vi "[FPGA] eHS Main (9039).vi"() -> ()   [LabVIEW 2017]
uses:
  <vilib>/OPAL-RT/eHS Toolkit/eHS Common/Controls/eHSx64 Gen3 Configuration.ctl
  <vilib>/OPAL-RT/Utilities Toolkit/Mapping/Input Mapping/FPGA/Controls/Input Mapping Configuration FIFO.ctl
  <vilib>/OPAL-RT/Utilities Toolkit/Mapping/Switch Mapping/FPGA/Controls/Switch Mapping Configuration FIFO.ctl
  <vilib>/OPAL-RT/Analog I-O Mapping & Conditioning Toolkit/AOMC/FPGA/Public/Controls/AOMC Configuration FIFO.ctl
  <vilib>/Platform/TimedLoop/XDataNode/timing_clust.ctl
  <vilib>/Platform/TimedLoop/XDataNode/nitl_modes.ctl
  <vilib>/Platform/TimedLoop/XDataNode/wakeup.ctl
  <vilib>/OPAL-RT/Analog I-O Mapping & Conditioning Toolkit/AIC/FPGA/Public/Controls/AIC Configuration FIFO.ctl
  <vilib>/OPAL-RT/FPGA Signal Generation Toolkit/Sinewave Generation/FPGA/Public/Controls/Sinewave Configuration FIFO.ctl
  <vilib>/OPAL-RT/FPGA Signal Generation Toolkit/SPWM Generation/FPGA/Public/Controls/SPWM Configuration FIFO.ctl
  <vilib>/OPAL-RT/FPGA Signal Generation Toolkit/PWM Generation/FPGA/Public/Controls/PWM Configuration FIFO.ctl
  <vilib>/OPAL-RT/Analog I-O Mapping & Conditioning Toolkit/AOMC/FPGA/Public/Controls/Input Sources.ctl
  <vilib>/OPAL-RT/Utilities Toolkit/Mapping/Input Mapping/FPGA/Controls/Sources/Input Sources - Parallelx32.ctl
  <vilib>/OPAL-RT/Utilities Toolkit/Mapping/Switch Mapping/FPGA/Controls/Sources/Switch Sources - Parallelx72.ctl
  <vilib>/rvi/Emulation/niFpgaGetClockAttributes.vi
  <vilib>/rvi/Emulation/niFpgaSctlEmulationGetInTimedLoop.vi
  <vilib>/rvi/Emulation/niFpgaEmulationReportErrorSimple.vi
  <vilib>/OPAL-RT/Utilities Toolkit/Mapping/Input Mapping/FPGA/SubVIs/Initialize/Initialize Input Mapping - Parallelx32.vi
  <vilib>/OPAL-RT/Utilities Toolkit/Mapping/Switch Mapping/FPGA/SubVIs/Initailize/Initialize Switch Mapping - Parallelx72.vi
  <vilib>/rvi/DataTransferAndStorage/Container/Common/niFpgaContainerExecOnDevCompGetState.vi
  <vilib>/rvi/Emulation/niFpgaEmulationIsFPGAContextNoSignature.vi
  <vilib>/rvi/DataTransferAndStorage/Container/Common/niFpgaContainerGetUniqueNameForEmu.vi
  <vilib>/rvi/Memory/Memory_Emulation/niFpgaMemoryEmulationCacheClearOnFirstRun.vi
  <vilib>/rvi/Memory/Memory_Emulation/nirvimemoryEmulationManagerCache_MakeExclusive.vi
  <vilib>/rvi/Memory/Memory_Emulation/niFpgaMemoryEmulationValidateCache.vi
  <vilib>/rvi/Memory/Memory_Emulation/nirvimemoryEmulationManagerCache_InsertValue.vi
  <vilib>/Utility/error.llb/Clear Errors.vi
  <vilib>/rvi/Memory/Memory_Emulation/nirvimemoryEmulationManagerCache_ReleaseExclusive.vi
  <vilib>/rvi/Memory/Memory_Emulation/nirvimemoryEmulationManagerCache_GetValue.vi
  <vilib>/rvi/Memory/Memory_Emulation/nirvimemoryEmulationManagerCache_SetValue.vi
  <vilib>/rvi/Emulation/niFpgaProcessEmulError.vi
  <vilib>/rvi/eio/common/nirviEmuTemplateMethod_errors.vi
  <vilib>/rvi/Emulation/niFpgaCriticalErrorInLSC.vi
  <vilib>/OPAL-RT/FPGA Signal Generation Toolkit/Sinewave Generation/FPGA/Private/Generators/Sinewave Generators (32-CH Parallel).vi
  <vilib>/OPAL-RT/FPGA Signal Generation Toolkit/SPWM Generation/FPGA/Private/Generators/SPWM Generators (12-CH Parallel).vi
  <vilib>/OPAL-RT/FPGA Signal Generation Toolkit/PWM Generation/FPGA/Private/Generators/PWM Generators (16-CH Parallel).vi
  <vilib>/OPAL-RT/Analog I-O Mapping & Conditioning Toolkit/AOMC/FPGA/Private/AO Mapping & Conditioning (FXP(20,5)).vi
  <vilib>/OPAL-RT/Analog I-O Mapping & Conditioning Toolkit/AIC/FPGA/Private/AI Conditioning FXP(20,5).vi
  <vilib>/OPAL-RT/eHS Toolkit/eHS FPGA/SubVIs/eHSx64 Gen3 Solver Core.vi
  <vilib>/OPAL-RT/Utilities Toolkit/Mapping/Switch Mapping/FPGA/SubVIs/Configure/Get Switch Mapping Configuration from Host - Parallelx72.vi
  <vilib>/OPAL-RT/Utilities Toolkit/Mapping/Input Mapping/FPGA/SubVIs/Configure/Get Input Mapping Configuration from Host - Parallelx32.vi
  <vilib>/OPAL-RT/Utilities Toolkit/Mapping/Switch Mapping/FPGA/SubVIs/Map/Map Switches - Parallelx72.vi
  <vilib>/OPAL-RT/Utilities Toolkit/Mapping/Input Mapping/FPGA/SubVIs/Map/Map Inputs - Parallelx32.vi
  <vilib>/rvi/interface/RandomDataEmulation/niFpgaRandomDataHandleErrors.vi
  <vilib>/Platform/TimedLoop/XDataNode/XDataNode.xnode
  <vilib>/rvi/DataTransferAndStorage/Container/XNode/niFpgaContainer.xnode
  <vilib>/rvi/DataTransferAndStorage/Register/Emulation/niFpgaRegisterEmulationRefIn.vi
  <vilib>/eio/EIONode/EIONode.xnode
  <vilib>/rvi/interface/RandomDataEmulation/nirviRandomDataFpgaReadWriteTemplate.vi
  <vilib>/Platform/TimedLoop/XDataNode/XDNodeRunTimeDep.lvlib
  <vilib>/OPAL-RT/Utilities Toolkit/Mapping/Input Mapping/FPGA/Input Mapping - FPGA.lvlib
  <vilib>/OPAL-RT/Utilities Toolkit/Mapping/Switch Mapping/FPGA/Switch Mapping - FPGA.lvlib
  <vilib>/OPAL-RT/Analog I-O Mapping & Conditioning Toolkit/AOMC/FPGA/AO Mapping & Conditioning - FPGA.lvlib
  <vilib>/OPAL-RT/Analog I-O Mapping & Conditioning Toolkit/AIC/FPGA/AI Conditioning - FPGA.lvlib
  <vilib>/OPAL-RT/eHS Toolkit/eHS FPGA/eHS - FPGA.lvlib
  <vilib>/OPAL-RT/Utilities Toolkit/Utilities/Type Casting/FPGA/Type Casting - FPGA.lvlib
  <vilib>/OPAL-RT/FPGA Signal Generation Toolkit/Sinewave Generation/FPGA/Sinewave Generation - FPGA.lvlib
  <vilib>/OPAL-RT/FPGA Signal Generation Toolkit/SPWM Generation/FPGA/SPWM Generation - FPGA.lvlib
  <vilib>/OPAL-RT/FPGA Signal Generation Toolkit/PWM Generation/FPGA/PWM Generation - FPGA.lvlib
  <vilib>/OPAL-RT/eHS Toolkit/eHS Common/eHS - Common.lvlib
panel:
  in  "View SPWM":bool
  in  "Mod Index":fxp<+/-,32,2>
  in  "Carrier Frequency":fxp<+/-,32,1>=0.00039999978616833687
  in  "Reset Sinewaves?":bool
  in  "Auto-Synchronize Sinewaves?":bool
  in  "Auto-Synchronize SPWM?":bool
  in  "Reset SPWMs?":bool
  in  "Reset PWMs?":bool
  out "Conditioned AI Data_Debug":sgl[](array[numeric])
  out "Mapped & Conditioned Data_Debug":fxp<+/-,20,5>[](array[numeric])
  in  "eHS Switches (CPU)":bool[](array[boolean])=[FALSE, FALSE, FALSE, FALSE, FALSE, FALSE, FALSE, FALSE, FALSE, FALSE, FALSE, FALSE, FALSE, FALSE, FALSE, FALSE, FALSE, FALSE, FALSE, FALSE, FALSE, FALSE, FALSE, FALSE, FALSE, FALSE, FALSE, FALSE, FALSE, FALSE, FALSE, FALSE, FALSE, FALSE, FALSE, FALSE, FALSE, FALSE, FALSE, FALSE, FALSE, FALSE, FALSE, FALSE, FALSE, FALSE, FALSE, FALSE, FALSE, FALSE, FALSE, FALSE, FALSE, FALSE, FALSE, FALSE, FALSE, FALSE, FALSE, FALSE, FALSE, FALSE, FALSE, FALSE, FALSE, FALSE, FALSE, FALSE, FALSE, FALSE, FALSE, FALSE]
  in  "eHS Input (CPU)":u32[](array[numeric])=[0, 0, 0, 0, 0, 0, 0, 0, 0, 0, 0, 0, 0, 0, 0, 0, 0, 0, 0, 0, 0, 0, 0, 0, 0, 0, 0, 0, 0, 0, 0, 0]
  in  "eHSx64 Gen3 Configuration":T1
  out "Finished":bool
  in  "stop":bool
  out "Module Underflow":bool
  out "Acq Loop Ticks":u32
  out "DMA FIFO Full":bool
  out "Chan Count":bool
  out "First Read":bool
  in  "Number of Channels":i32=4
  in  "Samps per Chan [Finite]":i32=5120
  in  "Acquisition Type":enum16{"Finite Samples", "Continuous Samples"}(ring)
  out "oclk div":u32
  out "oclk freq":u32
  in  "data rate (S/s)":u32
  out "oclk mult":u32
  out "FPGA Error":errorcluster
  in  "Chan Scale Array":sgl[](array[numeric])=[0.0, 0.0, 0.0, 0.0, 0.0, 0.0, 0.0, 0.0, 0.0, 0.0, 0.0, 0.0, 0.0, 0.0, 0.0, 0.0, 0.0, 0.0, 0.0, 0.0, 0.0, 0.0, 0.0, 0.0, 0.0, 0.0, 0.0, 0.0, 0.0, 0.0, 0.0, 0.0, 0.0, 0.0, 0.0, 0.0, 0.0, 0.0, 0.0, 0.0]
  # "Signal Generation Paramters"
  # "eHS Parameters"
  # "RIO Waveform Parameters"
  # "Debug"
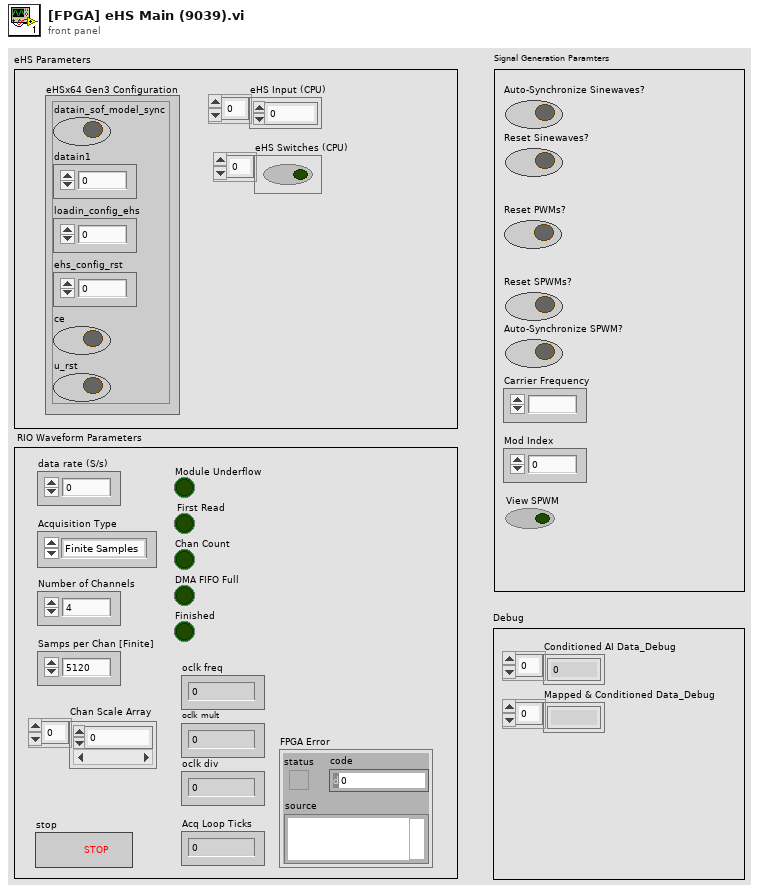
[diagram p1: front panel]
types:
  T1 = typedef "OPAL-RT eHS.lvlib/eHS - Common.lvlib/eHSx64 Gen3 Configuration.ctl" = cluster{"datain_sof_model_sync":bool, "datain1":fxp<+,33,33>, "loadin_config_ehs":fxp<+,33,33>, "ehs_config_rst":fxp<+,33,33>, "ce":bool, "u_rst":bool}
  T2 = typedef "PWM Generation - FPGA.lvlib/PWM Configuration FIFO.ctl" = refnum<k21>
  T3 = typedef "SPWM Generation - FPGA.lvlib/SPWM Configuration FIFO.ctl" = refnum<k21>
  T4 = typedef "Sinewave Generation - FPGA.lvlib/Sinewave Configuration FIFO.ctl" = refnum<k21>
  T5 = typedef "AI Conditioning - FPGA.lvlib/AIC Configuration FIFO.ctl" = refnum<k21>
  T6 = typedef "AO Mapping & Conditioning - FPGA.lvlib/AOMC Configuration FIFO.ctl" = refnum<k21>
  T7 = typedef "Switch Mapping - FPGA.lvlib/Switch Mapping Configuration FIFO.ctl" = refnum<k21>
  T8 = typedef "Input Mapping - FPGA.lvlib/Input Mapping Configuration FIFO.ctl" = refnum<k21>
  T9 = typedef "[FPGA] Local FPGA Memory.ctl" = cluster{"Analog Inputs":refnum<k21>, "Conditioned AI":refnum<k21>, "Analog Outputs (FXP(20,5))":refnum<k21>, "Analog Outputs (U16)":refnum<k21>, "Digital Inputs":refnum<k21>, "Digital Outputs":refnum<k21>, "eHS Outputs - Lane 1":refnum<k21>, "eHS Outputs - Lane 2":refnum<k21>, "eHS Outputs - Lane 3":refnum<k21>, "SWG Signals":refnum<k21>, "PWM Signals":refnum<k21>, "SPWM Signals":refnum<k21>}
  T10 = typedef "XDNodeRunTimeDep.lvlib/timing_clust.ctl" = cluster{"Expected End [f-1]":u64, "Actual End [f-1]":u64, "Finished Late? [f-1]":bool, "Expected End [i-1]":u64, "Actual End [i-1]":u64, "Finished Late? [i-1]":bool, "Expected Start [i]":u64, "Actual Start [i]":u64, "Expected Start [f]":u64, "Actual Start [f]":u64, "Source Name":string, "Structure Name":string, "Period":i64, "Deadline":i64, "Offset":i64, "Start":i64, "Priority":i32, "Timeout":i32, "Mode":T11, "Wakeup Reason":T12, "Error":errorcluster, "Source Type":string, "Secondary Source Type":string, "Global End Time":u64, "Global Start Time":u64, "Frame Duration":u64, "Iteration Duration":u64, "Assigned CPU":i32, "I/O Scan Engine Mode":u32}
  T11 = typedef "XDNodeRunTimeDep.lvlib/nitl_modes.ctl" = enum32{"No Change", "Process missed periods, maintain original phase", "Discard missed periods, maintain original phase", "Process missed periods, ignore original phase", "Discard missed periods, ignore original phase"}
  T12 = typedef "XDNodeRunTimeDep.lvlib/wakeup.ctl" = enum32{"Normal", "Aborted", "Asynchronous wakeup", "Timing source error", "Timed loop error", "Timeout"}
  T13 = typedef "Sinewave Generation - FPGA.lvlib/Sinewave Generator FPGA Resources.ctl" = cluster{"Sinewave Configuration FIFO":T4, "Sinewave Configuration Memory":T14}
  T14 = typedef "Sinewave Generation - FPGA.lvlib/Sinewave Generator Memory.ctl" = cluster{"Sinewave Generator Configuration Memory":cluster{"Sinewave Generator Configuration - Buffer 0":refnum<k21>, "Sinewave Generator Configuration - Buffer 1":refnum<k21>}, "Frequency Engine Rate Memory":T15, "Frequency Engine Values Memory":T16, "Sinewave LUT Memory":T17}
  T15 = typedef "Signal Generation Utilities - FPGA.lvlib/Frequency Engine Rate Memory.ctl" = cluster{"Frequency Engine Rates - Buffer 0":refnum<k21>, "Frequency Engine Rates - Buffer 1":refnum<k21>}
  T16 = typedef "Signal Generation Utilities - FPGA.lvlib/Frequency Engine Values Memory.ctl" = cluster{"Frequency Engine Values - Buffer 0":refnum<k21>, "Frequency Engine Values - Buffer 1":refnum<k21>}
  T17 = typedef "Signal Generation Utilities - FPGA.lvlib/Sinewave LUT Memory.ctl" = cluster{"Sinewave LUT (SGL)":refnum<k21>, "Sinewave LUT (16,1)":refnum<k21>}
  T18 = typedef "SPWM Generation - FPGA.lvlib/SPWM Generator FPGA Resources.ctl" = cluster{"SPWM Configuration FIFO":T3, "SPWM Generator Memory":T19}
  T19 = typedef "SPWM Generation - FPGA.lvlib/SPWM Generator Memory.ctl" = cluster{"SPWM Configuration Parameters Memory":T20, "Frequency Engine Rate Memory":T15, "Frequency Engine Values Memory":T16, "Sinewave LUT Memory":T17}
  T20 = typedef "SPWM Generation - FPGA.lvlib/SPWM Configuration Parameters Memory.ctl" = cluster{"SPWM Generator Configuration - Buffer 0":refnum<k21>, "SPWM Generator Configuration - Buffer 1":refnum<k21>}
  T21 = typedef "PWM Generation - FPGA.lvlib/PWM Generator FPGA Resources.ctl" = cluster{"PWM Generator Memory":T22, "PWM Configuration FIFO":T2}
  T22 = typedef "PWM Generation - FPGA.lvlib/PWM Generator Memory.ctl" = cluster{"PWM Generation Configuration":refnum<k21>, "PWM Generator States":refnum<k21>}
  T23 = typedef "Input Mapping - FPGA.lvlib/Input Mapping FPGA Resources.ctl" = cluster{"Input Mapping Configuration FIFO":T8, "Input Mapping Configuration Memory":T24}
  T24 = typedef "Input Mapping - FPGA.lvlib/Input Mapping Configuration Memory.ctl" = cluster{"Input Mapping Memory - Lane 0":refnum<k21>, "Input Mapping Memory - Lane 1":refnum<k21>, "Input Mapping Memory - Lane 2":refnum<k21>, "Input Mapping Memory - Lane 3":refnum<k21>}
  T25 = typedef "Switch Mapping - FPGA.lvlib/Switch Mapping FPGA Resources.ctl" = cluster{"Switch Mapping Configuration FIFO":T7, "Switch Mapping Configuration Memory":T26}
  T26 = typedef "Switch Mapping - FPGA.lvlib/Switch Mapping Configuration Memory.ctl" = cluster{"Switch Mapping Memory - Lane 0":refnum<k21>, "Switch Mapping Memory - Lane 1":refnum<k21>, "Switch Mapping Memory - Lane 2":refnum<k21>, "Switch Mapping Memory - Lane 3":refnum<k21>, "Switch Mapping Memory - Lane 4":refnum<k21>, "Switch Mapping Memory - Lane 5":refnum<k21>, "Switch Mapping Memory - Lane 6":refnum<k21>, "Switch Mapping Memory - Lane 7":refnum<k21>, "Switch Mapping Memory - Lane 8":refnum<k21>}
  T27 = typedef "AI Conditioning - FPGA.lvlib/AIC FPGA Resources.ctl" = cluster{"AIC Configuration FIFO":T5, "AIC Memory":T28}
  T28 = typedef "AI Conditioning - FPGA.lvlib/AIC Memory.ctl" = cluster{"AIC Configuration Parameters":refnum<k21>}
  T29 = typedef "AO Mapping & Conditioning - FPGA.lvlib/AOMC FPGA Resources.ctl" = cluster{"AOMC Memory":T30, "AOMC Configuration FIFO":T6}
  T30 = typedef "AO Mapping & Conditioning - FPGA.lvlib/AOMC Memory.ctl" = cluster{"AOMC Configuration Parameters":refnum<k21>}
  T31 = typedef "Sinewave Generation - FPGA.lvlib/Sinewave Generator Parameters.ctl" = cluster{"Number of Sinewaves to Generate":u8, "Read Buffer Index":u8, "Reset Sinewaves?":bool}
  T32 = typedef "SPWM Generation - FPGA.lvlib/SPWM FPGA Generator Parameters.ctl" = cluster{"Carrier Frequency":fxp<+/-,32,1>, "Mod Index ":fxp<+/-,32,2>, "Number of SPWMs to Generate":u8, "Reset SPWMs?":bool, "Read Buffer Index":u8}
  T33 = typedef "PWM Generation - FPGA.lvlib/PWM Generator Parameters.ctl" = cluster{"Number of PWMs to Generate":u8, "Reset PWMs?":bool}
  T34 = typedef "Switch Mapping - FPGA.lvlib/Switch Sources - Parallelx72.ctl" = cluster{"Group A":bool[], "Group B":bool[], "Group C":bool[], "Group D":bool[], "Group E":bool[]}
  T35 = typedef "Input Mapping - FPGA.lvlib/Input Sources - Parallelx32.ctl" = cluster{"Group A":u32[], "Group B":u32[], "Group C":u32[], "Group D":u32[]}
  T36 = typedef "AO Mapping & Conditioning - FPGA.lvlib/Input Sources.ctl" = cluster{"Group A":sgl[], "Group B":sgl[]}
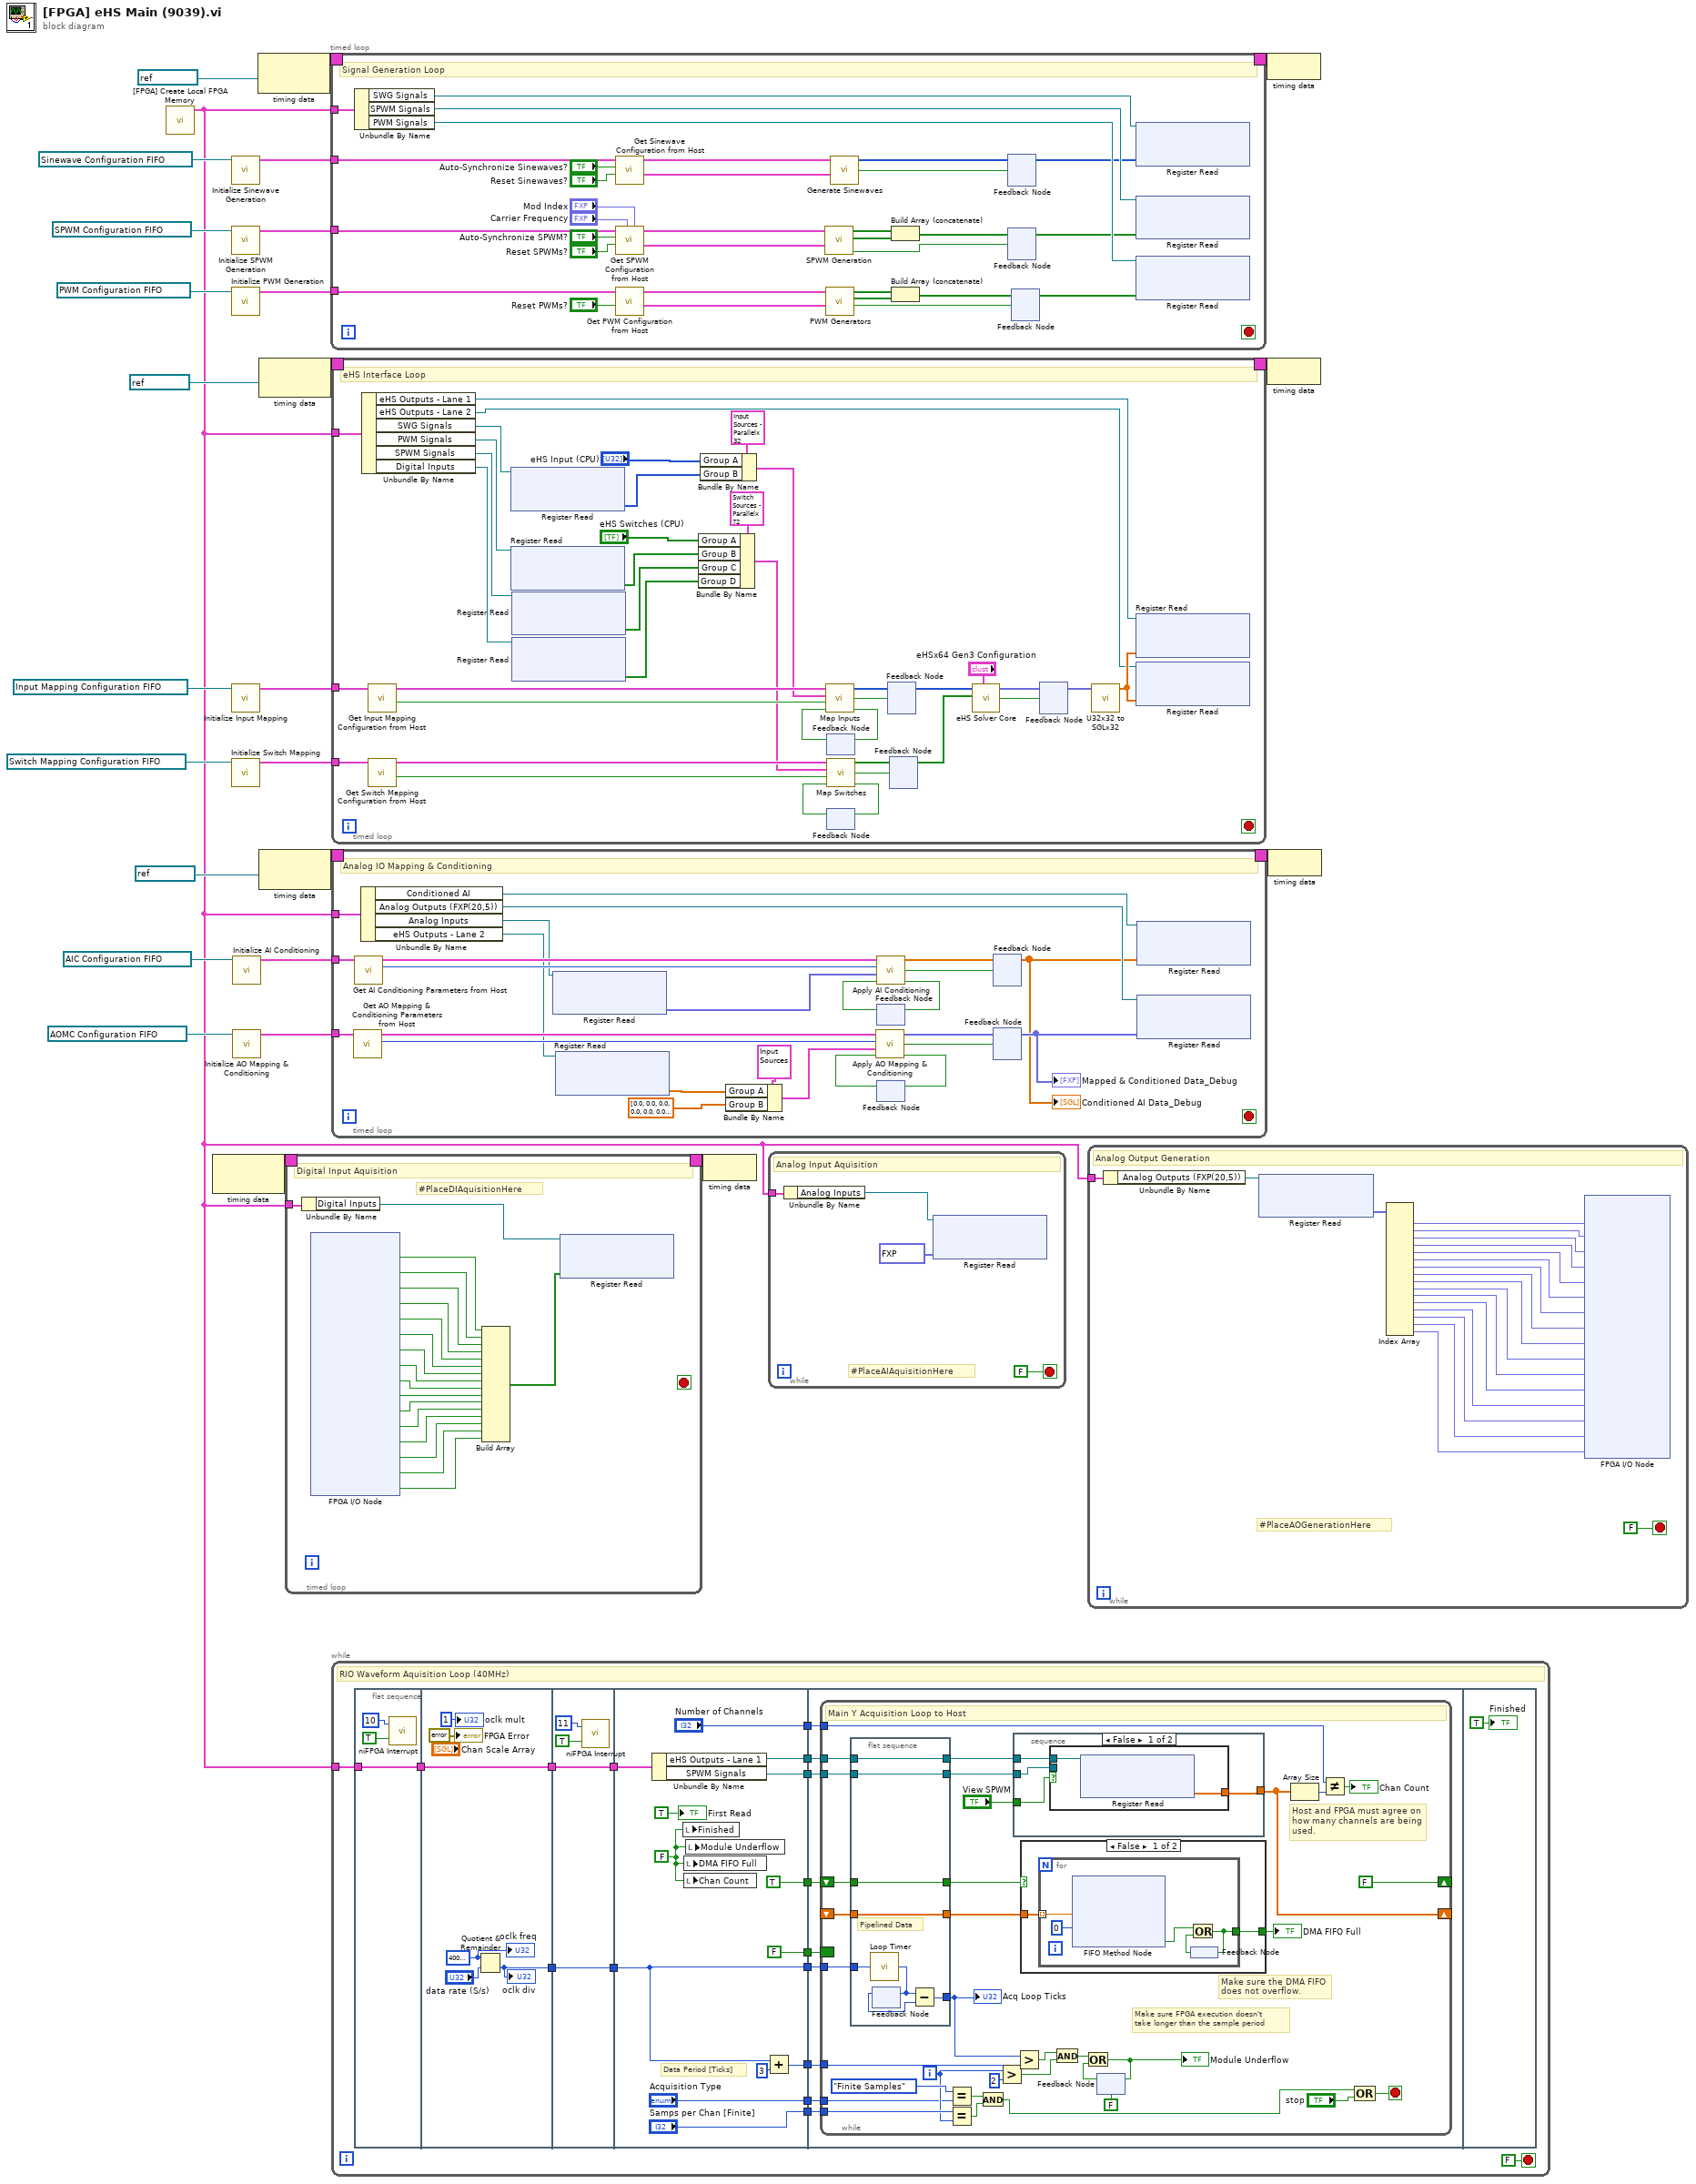
[diagram p0: block diagram]
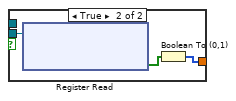
[diagram p2: hidden frame]
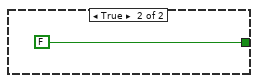
[diagram p3: hidden frame]
diagram:
  n1 = call "[FPGA] Create Local FPGA Memory.vi"() -> ("FPGA Memory"=w1:T9)  [unwired: 11 in]
  n2 = node-c288() -> (w3:T10)  [unwired: 1 in]
  n3 = call <vilib>:"Initialize Sinewave Generation.vi"("Sinewave Configuration FIFO"=T4 "Sinewave Configuration FIFO") -> ("Sinewave Generator FPGA Resources"=w4:T13)  [unwired: 10 in]
  n4 = call <vilib>:"Initialize SPWM Generation.vi"("SPWM Configuration FIFO"=T3 "SPWM Configuration FIFO") -> ("SPWM Generator FPGA Resources"=w5:T18)  [unwired: 10 in]
  n5 = call <vilib>:"Initialize PWM Generation.vi"("PWM Configuration FIFO"=T2 "PWM Configuration FIFO") -> ("PWM Generator FPGA Resources"=w6:T21)  [unwired: 10 in]
  n6 = call-poly <vilib>:"Initialize Input Mapping.vi"("Input Mapping Configuration FIFO"=T8 "Input Mapping Configuration FIFO") -> ("Input Mapping FPGA Resources"=w14:T23)  [unwired: 10 in]
  n7 = call-poly <vilib>:"Initialize Switch Mapping.vi"("Switch Mapping Configuration FIFO"=T7 "Switch Mapping Configuration FIFO") -> ("Switch Mapping FPGA Resources"=w13:T25)  [unwired: 10 in]
  n8 = call <vilib>:"Initialize AI Conditioning.vi"("AIC Configuration FIFO"=T5 "AIC Configuration FIFO") -> ("AIC FPGA Resources"=w16:T27)  [unwired: 10 in]
  n9 = call <vilib>:"Initialize AO Mapping & Conditioning.vi"("AOMC Configuration FIFO"=T6 "AOMC Configuration FIFO") -> ("AOMC FPGA Resources"=w15:T29)  [unwired: 10 in]
  n10 = node-c288(refnum<k21> "100MHz" ("Source Name")) -> (w12:T10)
  n11 = node-c288(refnum<k21> "200MHz" ("Source Name")) -> (w26:T10)
  n12 = node-c288(refnum<k21> "200MHz" ("Source Name")) -> (w20:T10)
  n13 = timed-loop {
    timing: w3 -> [_]
    timing-out: [_] -> w2
    tunnel: w1 -> [w45]
    stop <- _ stop-if-true
    # "#PlaceDIAquisitionHere"
    # "Digital Input Aquisition"
    n14 = Unbundle By Name(w45) -> ("Digital Inputs"=w44:refnum<k21>)
    n15 = xnode "FPGA I/O Node"() -> ("Mod3/DIO0"=w43:bool, "Mod3/DIO1"=w42:bool, "Mod3/DIO2"=w41:bool, "Mod3/DIO3"=w40:bool, "Mod3/DIO4"=w39:bool, "Mod3/DIO5"=w38:bool, "Mod3/DIO6"=w37:bool, "Mod3/DIO7"=w36:bool, "Mod4/DIO0"=w35:bool, "Mod4/DIO1"=w34:bool, "Mod4/DIO2"=w33:bool, "Mod4/DIO3"=w32:bool, "Mod4/DIO4"=w31:bool, "Mod4/DIO5"=w30:bool, "Mod4/DIO6"=w29:bool, "Mod4/DIO7"=w28:bool)  [unwired: 16 in, 16 out]
    n16 = Build Array(w43, w42, w41, w40, w39, w38, w37, w36, w35, w34, w33, w32, w31, w30, w29, w28) -> (w27:bool[])
    n17 = xnode ("Register Read")("Data"=w27, "Register In"=w44) -> ()  [unwired: 1 out]
  }
  n18 = timed-loop {
    timing: w12 -> [_]
    timing-out: [_] -> w11
    tunnel: w1 -> [w80]
    tunnel: w6 -> [w79]
    tunnel: w5 -> [w78]
    tunnel: w4 -> [w77]
    stop <- _ stop-if-true
    # "Signal Generation Loop"
    n19 = Unbundle By Name(w80) -> ("SWG Signals"=w63:refnum<k21>, "SPWM Signals"=w62:refnum<k21>, "PWM Signals"=w61:refnum<k21>)
    n20 = call <vilib>:"Get Sinewave Configuration from Host.vi"("Reset Sinewaves?"="Reset Sinewaves?", "Auto-Synchronize Sinewaves?"="Auto-Synchronize Sinewaves?", "Sinewave Generator FPGA Resources"=w77) -> ("Sinewave Generator Parameters"=w70:T31, "Sinewave Configuration Memory"=w71:T14)  [unwired: 7 in]
    n21 = call <vilib>:"Get SPWM Configuration from Host.vi"("Mod Index"="Mod Index", "Carrier Frequency"="Carrier Frequency", "Reset SPWMs?"="Reset SPWMs?", "Auto-Synchronize SPWM?"="Auto-Synchronize SPWM?", "SPWM Generator FPGA Resources"=w78) -> ("SPWM Generator Parameters"=w68:T32, "SPWM Generator Memory"=w69:T19)  [unwired: 5 in]
    n22 = call <vilib>:"Get PWM Configuration from Host.vi"("Reset PWMs?"="Reset PWMs?", "PWM Generator FPGA Resources"=w79) -> ("PWM Generator Parameters"=w66:T33, "PWM Generator Memory"=w67:T22)  [unwired: 8 in]
    n23 = call-poly <vilib>:"SPWM Generation.vi"("SPWM Generator Parameters"=w68, "SPWM Generator Memory"=w69) -> ("Output Valid"=w51:bool, "!SPWM States"=w56:bool[], "SPWM States"=w57:bool[])  [unwired: 7 in]
    n24 = call-poly <vilib>:"PWM Generators.vi"("PWM Generator Parameters"=w66, "PWM Generator Memory"=w67) -> ("Output Valid?"=w49:bool, "!PWM States"=w52:bool[], "PWM States"=w53:bool[])  [unwired: 7 in]
    n25 = call-poly <vilib>:"Generate Sinewaves.vi"("Sinewave Generator Parameters"=w70, "Sinewave Generator Memory"=w71) -> ("Output Valid?"=w59:bool, "Sinewave (SGL-as-U32)"=w60:u32[])  [unwired: 8 in]
    n26 = Build Array (concatenate)(w57, w56) -> (w55:bool[])
    n27 = Build Array (concatenate)(w53, w52) -> (w50:bool[])
    n28 = feedback-in #1(w60, w59) -> ()
    n29 = feedback #1() -> (w58:u32[])  [unwired: 1 in]
    n30 = feedback #2() -> (w54:bool[])  [unwired: 1 in]
    n31 = feedback-in #2(w55, w51) -> ()
    n32 = feedback #3() -> (w48:bool[])  [unwired: 1 in]
    n33 = feedback-in #3(w50, w49) -> ()
    n34 = xnode ("Register Read")("Data"=w58, "Register In"=w63) -> ()  [unwired: 1 out]
    n35 = xnode ("Register Read")("Data"=w54, "Register In"=w62) -> ()  [unwired: 1 out]
    n36 = xnode ("Register Read")("Data"=w48, "Register In"=w61) -> ()  [unwired: 1 out]
  }
  n37 = timed-loop {
    timing: w26 -> [_]
    timing-out: [_] -> w25
    tunnel: w1 -> [w99]
    tunnel: w14 -> [w119]
    tunnel: w13 -> [w117]
    stop <- _ stop-if-true
    # "eHS Interface Loop"
    n38 = Unbundle By Name(w99) -> ("eHS Outputs - Lane 1"=w94:refnum<k21>, "eHS Outputs - Lane 2"=w91:refnum<k21>, "SWG Signals"=w90:refnum<k21>, "PWM Signals"=w89:refnum<k21>, "SPWM Signals"=w88:refnum<k21>, "Digital Inputs"=w84:refnum<k21>)
    n39 = call-poly <vilib>:"Get Input Mapping Configuration from Host.vi"("Input Mapping FPGA Resources"=w119) -> ("Settings Updated?"=w110:bool, "Input Mapping Configuration Memory"=w118:T24)  [unwired: 9 in]
    n40 = call-poly <vilib>:"Get Switch Mapping Configuration from Host.vi"("Switch Mapping FPGA Resources"=w117) -> ("Settings Updated?"=w111:bool, "Switch Mapping Configuration Memory"=w112:T26)  [unwired: 9 in]
    n41 = xnode ("Register Read")("Register In"=w90) -> ("Data"=w87:u32[])  [unwired: 1 out]
    n42 = xnode ("Register Read")("Register In"=w89) -> ("Data"=w86:bool[])  [unwired: 1 out]
    n43 = xnode ("Register Read")("Register In"=w88) -> ("Data"=w85:bool[])  [unwired: 1 out]
    n44 = xnode ("Register Read")("Register In"=w84) -> ("Data"=w83:bool[])  [unwired: 1 out]
    n45 = Bundle By Name(cluster=T34 {"Group A"=[FALSE, FALSE, FALSE, FALSE, FALSE, FALSE, FALSE, FALSE, FALSE, FALSE, FALSE, FALSE, FALSE, FALSE, FALSE, FALSE, FALSE, FALSE, FALSE, FALSE, FALSE, FALSE, FALSE, FALSE, FALSE, FALSE, FALSE, FALSE, FALSE, FALSE, FALSE, FALSE, FALSE, FALSE, FALSE, FALSE, FALSE, FALSE, FALSE, FALSE, FALSE, FALSE, FALSE, FALSE, FALSE, FALSE, FALSE, FALSE, FALSE, FALSE, FALSE, FALSE, FALSE, FALSE, FALSE, FALSE, FALSE, FALSE, FALSE, FALSE, FALSE, FALSE, FALSE, FALSE, FALSE, FALSE, FALSE, FALSE, FALSE, FALSE, FALSE, FALSE], "Group B"=[FALSE, FALSE, FALSE, FALSE, FALSE, FALSE, FALSE, FALSE, FALSE, FALSE, FALSE, FALSE, FALSE, FALSE, FALSE, FALSE, FALSE, FALSE, FALSE, FALSE, FALSE, FALSE, FALSE, FALSE, FALSE, FALSE, FALSE, FALSE, FALSE, FALSE, FALSE, FALSE, FALSE, FALSE, FALSE, FALSE, FALSE, FALSE, FALSE, FALSE, FALSE, FALSE, FALSE, FALSE, FALSE, FALSE, FALSE, FALSE, FALSE, FALSE, FALSE, FALSE, FALSE, FALSE, FALSE, FALSE, FALSE, FALSE, FALSE, FALSE, FALSE, FALSE, FALSE, FALSE, FALSE, FALSE, FALSE, FALSE, FALSE, FALSE, FALSE, FALSE], "Group C"=[FALSE, FALSE, FALSE, FALSE, FALSE, FALSE, FALSE, FALSE, FALSE, FALSE, FALSE, FALSE, FALSE, FALSE, FALSE, FALSE, FALSE, FALSE, FALSE, FALSE, FALSE, FALSE, FALSE, FALSE, FALSE, FALSE, FALSE, FALSE, FALSE, FALSE, FALSE, FALSE, FALSE, FALSE, FALSE, FALSE, FALSE, FALSE, FALSE, FALSE, FALSE, FALSE, FALSE, FALSE, FALSE, FALSE, FALSE, FALSE, FALSE, FALSE, FALSE, FALSE, FALSE, FALSE, FALSE, FALSE, FALSE, FALSE, FALSE, FALSE, FALSE, FALSE, FALSE, FALSE, FALSE, FALSE, FALSE, FALSE, FALSE, FALSE, FALSE, FALSE], "Group D"=[FALSE, FALSE, FALSE, FALSE, FALSE, FALSE, FALSE, FALSE, FALSE, FALSE, FALSE, FALSE, FALSE, FALSE, FALSE, FALSE, FALSE, FALSE, FALSE, FALSE, FALSE, FALSE, FALSE, FALSE, FALSE, FALSE, FALSE, FALSE, FALSE, FALSE, FALSE, FALSE, FALSE, FALSE, FALSE, FALSE, FALSE, FALSE, FALSE, FALSE, FALSE, FALSE, FALSE, FALSE, FALSE, FALSE, FALSE, FALSE, FALSE, FALSE, FALSE, FALSE, FALSE, FALSE, FALSE, FALSE, FALSE, FALSE, FALSE, FALSE, FALSE, FALSE, FALSE, FALSE, FALSE, FALSE, FALSE, FALSE, FALSE, FALSE, FALSE, FALSE], "Group E"=[FALSE, FALSE, FALSE, FALSE, FALSE, FALSE, FALSE, FALSE, FALSE, FALSE, FALSE, FALSE, FALSE, FALSE, FALSE, FALSE, FALSE, FALSE, FALSE, FALSE, FALSE, FALSE, FALSE, FALSE, FALSE, FALSE, FALSE, FALSE, FALSE, FALSE, FALSE, FALSE, FALSE, FALSE, FALSE, FALSE, FALSE, FALSE, FALSE, FALSE, FALSE, FALSE, FALSE, FALSE, FALSE, FALSE, FALSE, FALSE, FALSE, FALSE, FALSE, FALSE, FALSE, FALSE, FALSE, FALSE, FALSE, FALSE, FALSE, FALSE, FALSE, FALSE, FALSE, FALSE, FALSE, FALSE, FALSE, FALSE, FALSE, FALSE, FALSE, FALSE]} ("Switch Sources"), "Group A"="eHS Switches (CPU)", "Group B"=w86, "Group C"=w85, "Group D"=w83) -> (w107:T34)
    n46 = Bundle By Name(cluster=T35 {"Group A"=[0, 0, 0, 0, 0, 0, 0, 0, 0, 0, 0, 0, 0, 0, 0, 0, 0, 0, 0, 0, 0, 0, 0, 0, 0, 0, 0, 0, 0, 0, 0, 0], "Group B"=[0, 0, 0, 0, 0, 0, 0, 0, 0, 0, 0, 0, 0, 0, 0, 0, 0, 0, 0, 0, 0, 0, 0, 0, 0, 0, 0, 0, 0, 0, 0, 0], "Group C"=[0, 0, 0, 0, 0, 0, 0, 0, 0, 0, 0, 0, 0, 0, 0, 0, 0, 0, 0, 0, 0, 0, 0, 0, 0, 0, 0, 0, 0, 0, 0, 0], "Group D"=[0, 0, 0, 0, 0, 0, 0, 0, 0, 0, 0, 0, 0, 0, 0, 0, 0, 0, 0, 0, 0, 0, 0, 0, 0, 0, 0, 0, 0, 0, 0, 0]} ("Input Sources"), "Group A"="eHS Input (CPU)", "Group B"=w87) -> (w106:T35)
    n47 = feedback #4() -> (w115:bool)  [unwired: 1 in]
    n48 = call-poly <vilib>:"Map Inputs.vi"("Input Valid?"=w115, "Settings Updated?"=w110, "Input Sources"=w106, "Input Mapping Configuration Memory"=w118) -> ("Ready for Input?"=w116:bool, "Output Valid?"=w105:bool, "Mapped Inputs"=w104:u32[])  [unwired: 5 in]
    n49 = feedback-in #4(w116) -> ()
    n50 = feedback #5() -> (w113:bool)  [unwired: 1 in]
    n51 = call-poly <vilib>:"Map Switches.vi"("Input Valid?"=w113, "Settings Updated?"=w111, "Switch Sources"=w107, "Switch Mapping Configuration Memory"=w112) -> ("Ready for Input?"=w114:bool, "Output Valid?"=w103:bool, "Mapped Switches"=w102:bool[])  [unwired: 5 in]
    n52 = feedback-in #5(w114) -> ()
    n53 = feedback #6() -> (w100:u32[])  [unwired: 1 in]
    n54 = feedback-in #6(w104, w105) -> ()
    n55 = feedback #7() -> (w101:bool[])  [unwired: 1 in]
    n56 = feedback-in #7(w102, w103) -> ()
    n57 = call-poly <vilib>:"eHS Solver Core.vi"("eHSx64 Gen3 Configuration"="eHSx64 Gen3 Configuration", "eHSx64 Switches (SW)"=w101, "eHSx64 Inputs (U)"=w100) -> ("Output Valid?"=w96:bool, "eHSx64 Outputs (Y)"=w95:fxp<+,32,32>[])  [unwired: 5 in, 2 out]
    n58 = feedback #8() -> (w93:fxp<+,32,32>[])  [unwired: 1 in]
    n59 = feedback-in #8(w95, w96) -> ()
    n60 = call <vilib>:"U32x32 to SGLx32.vi"("U32x32"=w93) -> ("SGLx32"=w92:sgl[])  [unwired: 10 in]
    n61 = xnode ("Register Read")("Data"=w92, "Register In"=w94) -> ()  [unwired: 1 out]
    n62 = xnode ("Register Read")("Data"=w92, "Register In"=w91) -> ()  [unwired: 1 out]
  }
  n63 = timed-loop {
    timing: w20 -> [_]
    timing-out: [_] -> w19
    tunnel: w1 -> [w142]
    tunnel: w16 -> [w146]
    tunnel: w15 -> [w145]
    stop <- _ stop-if-true
    # "Analog IO Mapping & Conditioning"
    n64 = call <vilib>:"Get AO Mapping & Conditioning Parameters from Host.vi"("AOMC FPGA Resources"=w145) -> ("Number of Active AO Channels"=w143:u8, "AOMC Memory"=w144:T30)  [unwired: 9 in]
    n65 = call <vilib>:"Get AI Conditioning Parameters from Host.vi"("AIC FPGA Resources"=w146) -> ("Number of Active AI Channels"=w148:u8, "AIC Memory"=w147:T28)  [unwired: 9 in]
    n66 = Unbundle By Name(w142) -> ("Conditioned AI"=w132:refnum<k21>, "Analog Outputs (FXP(20,5))"=w131:refnum<k21>, "Analog Inputs"=w134:refnum<k21>, "eHS Outputs - Lane 2"=w141:refnum<k21>)
    n67 = xnode ("Register Read")("Register In"=w134) -> ("Data"=w133:fxp<+/-,20,5>[])  [unwired: 1 out]
    n68 = xnode ("Register Read")("Register In"=w141) -> ("Data"=w125:sgl[])  [unwired: 1 out]
    n69 = Bundle By Name(cluster=T36 {"Group A"=[0.0, 0.0, 0.0, 0.0, 0.0, 0.0, 0.0, 0.0, 0.0, 0.0, 0.0, 0.0, 0.0, 0.0, 0.0, 0.0, 0.0, 0.0, 0.0, 0.0, 0.0, 0.0, 0.0, 0.0, 0.0, 0.0, 0.0, 0.0, 0.0, 0.0, 0.0, 0.0], "Group B"=[0.0, 0.0, 0.0, 0.0, 0.0, 0.0, 0.0, 0.0, 0.0, 0.0, 0.0, 0.0, 0.0, 0.0, 0.0, 0.0, 0.0, 0.0, 0.0, 0.0, 0.0, 0.0, 0.0, 0.0, 0.0, 0.0, 0.0, 0.0, 0.0, 0.0, 0.0, 0.0]} ("Solver Data"), "Group A"=w125, "Group B"=sgl[] [0.0, 0.0, 0.0, 0.0, 0.0, 0.0, 0.0, 0.0, 0.0, 0.0, 0.0, 0.0, 0.0, 0.0, 0.0, 0.0, 0.0, 0.0, 0.0, 0.0, 0.0, 0.0, 0.0, 0.0, 0.0, 0.0, 0.0, 0.0, 0.0, 0.0, 0.0, 0.0]) -> (w135:T36)
    n70 = feedback #9() -> (w139:bool)  [unwired: 1 in]
    n71 = call-poly <vilib>:"Apply AI Conditioning.vi"("Input Valid?"=w139, "AI Data"=w133, "Number of Supported AI Channels"=w148, "AIC Memory"=w147) -> ("Ready for Input?"=w140:bool, "Output Valid?"=w130:bool, "Conditioned AI Data"=w129:sgl[])  [unwired: 5 in]
    n72 = feedback-in #9(w140) -> ()
    n73 = feedback #10() -> (w137:bool)  [unwired: 1 in]
    n74 = call-poly <vilib>:"Apply AO Mapping & Conditioning.vi"("Input Valid?"=w137, "Data"=w135, "Number of Active AO Channels"=w143, "AOMC Memory"=w144) -> ("Ready for Input?"=w138:bool, "Output Valid?"=w127:bool, "Mapped & Conditioned Data"=w128:fxp<+/-,20,5>[])  [unwired: 5 in]
    n75 = feedback-in #10(w138) -> ()
    n76 = feedback #11() -> (w123:sgl[])  [unwired: 1 in]
    "Conditioned AI Data_Debug" <- w123
    n77 = feedback-in #11(w129, w130) -> ()
    n78 = feedback #12() -> (w126:fxp<+/-,20,5>[])  [unwired: 1 in]
    "Mapped & Conditioned Data_Debug" <- w126
    n79 = feedback-in #12(w128, w127) -> ()
    n80 = xnode ("Register Read")("Data"=w123, "Register In"=w132) -> ()  [unwired: 1 out]
    n81 = xnode ("Register Read")("Data"=w126, "Register In"=w131) -> ()  [unwired: 1 out]
  }
  n82 = while {
    tunnel: w1 -> [w155]
    stop <- FALSE stop-if-true
    # "RIO Waveform Aquisition Loop (40MHz)"
    n83 = flat-sequence {
      tunnel: w155 -> [w167]
      tunnel: [w167] -> w154
      tunnel: [w173] -> w160
      tunnel: w154 -> [w172]
      tunnel: [w172] -> w153
      tunnel: [w177] -> w161
      tunnel: w160 -> [w177]
      tunnel: [w176] -> w156
      tunnel: w153 -> [w176]
      tunnel: ["Number of Channels"] -> w166
      tunnel: ["Samps per Chan [Finite]"] -> w165
      tunnel: [w186] -> w164
      tunnel: [w187] -> w163
      tunnel: [TRUE] -> w162
      tunnel: w161 -> [w186]
      tunnel: [FALSE] -> w159
      tunnel: ["Acquisition Type"] -> w157
      tunnel: w156 -> [w182]
      tunnel: [w181] -> w152
      tunnel: [w180] -> w151
      tunnel: w166 -> [w201]
      tunnel: w165 -> [w199]
      tunnel: w164 -> [w200]
      tunnel: w163 -> [w198]
      tunnel: w162 -> [w197]
      tunnel: w159 -> [w196]
      tunnel: w157 -> [w195]
      tunnel: w152 -> [w194]
      tunnel: w151 -> [w193]
      frame #0 {
        n84 = call <vilib>:"niFPGA Interrupt.vi"("Wait Until Cleared (F)"=TRUE ("Wait Until Cleared"), "IRQ Number (0)"=u8 10 ("IRQ Number")) -> ()  [unwired: 1 in]
      }
      frame #1 {
        w174 = u32 40000000 ("oclk freq")
        n85 = Quotient & Remainder(x=w174, y="data rate (S/s)") -> (floor(x/y)=w173:u32)  [unwired: 1 out]
        "oclk div" <- w173
        "oclk freq" <- w174
        "oclk mult" <- u32 1 ("oclk mult")
        "FPGA Error" <- errorcluster {"status"=FALSE, "code"=0, "source"=""} ("FPGA Error")
      }
      frame #2 {
        n86 = call <vilib>:"niFPGA Interrupt.vi"("Wait Until Cleared (F)"=TRUE ("Wait Until Cleared"), "IRQ Number (0)"=u8 11 ("IRQ Number")) -> ()  [unwired: 1 in]
      }
      frame #3 {
        w191 = FALSE ("Module Underflow")
        # "Data Period [Ticks]"
        n87 = Unbundle By Name(w182) -> ("eHS Outputs - Lane 1"=w181:refnum<k21>, "SPWM Signals"=w180:refnum<k21>)
        n88 = local write "Finished"(w191) -> ()
        n89 = local write "DMA FIFO Full"(w191) -> ()
        n90 = local write "Chan Count"(w191) -> ()
        n91 = local write "Module Underflow"(w191) -> ()
        n92 = Add(x=w186, y=u32 3) -> (x+y=w187:u32)
        "First Read" <- TRUE ("First Read")
      }
      frame #4 {
        n93 = while {
          tunnel: w199 -> [w230]
          shift-right: [w215] -> _
          shift-left: _ -> [w225]
          tunnel: w201 -> [w208]
          tunnel: w200 -> [w229]
          tunnel: w198 -> [w227]
          shift-right: [FALSE] -> _
          shift-left: w197 -> [w211]
          border: w196 -> [_]
          tunnel: w195 -> [w213]
          tunnel: w194 -> [w209]
          tunnel: w193 -> [w203]
          i -> [w223]
          stop <- w233 stop-if-true
          # "Host and FPGA must agree on \nhow many channels are being\nused."
          # "Make sure the DMA FIFO\ndoes not overflow."
          # "Make sure FPGA execution doesn't\ntake longer than the sample period"
          # "Main Y Acquisition Loop to Host"
          n94 = flat-sequence {
            tunnel: w229 -> [w260]
            tunnel: [w257] -> w226
            tunnel: [w256] -> w214
            tunnel: w225 -> [w256]
            tunnel: [w255] -> w212
            tunnel: w211 -> [w255]
            tunnel: [w254] -> w210
            tunnel: w209 -> [w254]
            tunnel: [w253] -> w204
            tunnel: w203 -> [w253]
            frame #0 {
              # "Pipelined Data"
              n95 = call "Loop Timer"("Count(Ticks)"=w260) -> ("Tick Count(Ticks)"=w258:u32)
              n96 = feedback-in #13(w258) -> ()
              n97 = feedback #13() -> (w259:u32)  [unwired: 1 out]
              n98 = Subtract(x=w258, y=w259) -> (x-y=w257:u32)
            }
          }
          n99 = Equal?(x=enum16{"Finite Samples", "Continuous Samples"}."Finite Samples" ("y"), y=w213) -> (x = y?=w218:bool)
          n100 = Equal?(x=w230, y=w223) -> (x = y?=w217:bool)
          n101 = And(x=w218, y=w217) -> (x .and. y?=w216:bool)
          n102 = Greater?(x=w223, y=2) -> (0:w205:bool)
          n103 = stacked-sequence {
            tunnel: [w238] -> w215
            tunnel: w210 -> [w239]
            tunnel: w204 -> [w236]
            tunnel: "View SPWM" -> [w237]
            frame #0 {
              n104 = case shown="False" w237 {
                tunnel: w239 -> [w241 _]
                tunnel: [w240 w242] -> w238
                tunnel: w236 -> [_ w244]
                frame False {
                  n105 = xnode ("Register Read")("Register In"=w241) -> ("Data"=w240:sgl[])  [unwired: 1 out]
                }
                frame True {
                  n106 = xnode ("Register Read")("Register In"=w244) -> ("Data"=w243:bool[])  [unwired: 1 out]
                  n107 = Boolean To (0,1)(Boolean=w243) -> (0, 1=w242:i16[])
                }
              }
            }
          }
          n108 = Greater?(x=w226, y=w227) -> (0:w206:bool)
          n109 = case shown="False" w212 {
            tunnel: [w246 FALSE] -> w232
            tunnel: w214 -> [w245 _]
            frame False {
              n110 = for {
                tunnel: [w250] -> w246
                tunnel: w245 -> [w247] mode=indexing
                n111 = xnode ("FIFO Method Node")("Element"=w247, "Timeout"=0) -> ("Timed Out?"=w248:bool)  [unwired: 1 in, 1 out]
                n112 = feedback #14() -> (w251:bool)
                n113 = Or(x=w248, y=w251) -> (x .or. y?=w250:bool)
                n114 = feedback-in #14(w250) -> ()
              }
            }
            frame True {
            }
          }
          "DMA FIFO Full" <- w232
          n115 = And(x=w206, y=w205) -> (x .and. y?=w220:bool)
          n116 = feedback #15(FALSE) -> (w222:bool)
          n117 = Or(x=w220, y=w222) -> (x .or. y?=w219:bool)
          "Module Underflow" <- w219
          n118 = feedback-in #15(w219) -> ()
          n119 = Array Size(array=w215) -> (size(s)=w207:i32)
          n120 = Not Equal?(x=w208, y=w207) -> (x != y?=→"Chan Count":bool)
          n121 = Compound Arithmetic op=OR(w216, "stop") -> (w233:bool)
          "Acq Loop Ticks" <- w226
        }
      }
      frame #5 {
        "Finished" <- TRUE ("Finished")
      }
    }
  }
  n122 = node-c288(w2) -> ()
  n123 = while {
    tunnel: w1 -> [w264]
    stop <- FALSE stop-if-true
    # "#PlaceAIAquisitionHere"
    # "Analog Input Aquisition"
    n124 = Unbundle By Name(w264) -> ("Analog Inputs"=w263:refnum<k21>)
    n125 = xnode ("Register Read")("Data"=fxp<+/-,20,5>[] [0.0, 0.0, 0.0, 0.0, 0.0, 0.0, 0.0, 0.0, 0.0, 0.0, 0.0, 0.0, 0.0, 0.0, 0.0, 0.0, 0.0, 0.0, 0.0, 0.0, 0.0, 0.0, 0.0, 0.0, 0.0, 0.0, 0.0, 0.0, 0.0, 0.0, 0.0, 0.0], "Register In"=w263) -> ()  [unwired: 1 out]
  }
  n126 = while {
    tunnel: w1 -> [w284]
    stop <- FALSE stop-if-true
    # "#PlaceAOGenerationHere"
    # "Analog Output Generation"
    n127 = Unbundle By Name(w284) -> ("Analog Outputs (FXP(20,5))"=w283:refnum<k21>)
    n128 = xnode ("Register Read")("Register In"=w283) -> ("Data"=w282:fxp<+/-,20,5>[])  [unwired: 1 out]
    n129 = Index Array(array=w282) -> (element #1=w281:fxp<+/-,20,5>, element #2=w280:fxp<+/-,20,5>, element #3=w279:fxp<+/-,20,5>, element #4=w278:fxp<+/-,20,5>, element #5=w277:fxp<+/-,20,5>, element #6=w276:fxp<+/-,20,5>, element #7=w275:fxp<+/-,20,5>, element #8=w274:fxp<+/-,20,5>, element #9=w273:fxp<+/-,20,5>, element #10=w272:fxp<+/-,20,5>, element #11=w271:fxp<+/-,20,5>, element #12=w270:fxp<+/-,20,5>, element #13=w269:fxp<+/-,20,5>, element #14=w268:fxp<+/-,20,5>, element #15=w267:fxp<+/-,20,5>, element #16=w266:fxp<+/-,20,5>)  [unwired: 16 in]
    n130 = xnode "FPGA I/O Node"("Mod2/AO0"=w281, "Mod2/AO1"=w280, "Mod2/AO2"=w279, "Mod2/AO3"=w278, "Mod5/AO0"=w277, "Mod5/AO1"=w276, "Mod5/AO2"=w275, "Mod5/AO3"=w274, "Mod6/AO0"=w273, "Mod6/AO1"=w272, "Mod6/AO2"=w271, "Mod6/AO3"=w270, "Mod7/AO0"=w269, "Mod7/AO1"=w268, "Mod7/AO2"=w267, "Mod7/AO3"=w266) -> ()  [unwired: 16 in, 16 out]
  }
  n131 = node-c288(w11) -> ()
  n132 = node-c288(w25) -> ()
  n133 = node-c288(w19) -> ()
